vi "Set Exclusions.vi"(4 "Exclude dependent shared libraries":bool, 6 "Exclude dependent packed libraries":bool, 8 "error in (no error)":errorcluster, 9 "Disconnect inline subVIs (T)":bool=TRUE, 10 "Exclusions":T1={"Disconnect type definitions"=FALSE, "Remove unused polymorphic VI instances"=TRUE, "Remove unused members of project libraries"=TRUE, "Modify project library file after removing unused members"=TRUE}, 11 "DLL in":refnum<class "NI_AB_API_DLL.lvclass">) -> (0 "error out":errorcluster, 3 "DLL out":refnum<class "NI_AB_API_DLL.lvclass">)   [LabVIEW 2020, in "NI_AB_API_DLL.lvclass"]
uses:
  <vilib>/AppBuilder/AB_API/DLL/NI_AB_API_DLL.lvclass
  <vilib>/AppBuilder/AB_API/common/AB_API Primary Exclusions.ctl
  <vilib>/AppBuilder/AB_API/Application/NI_AB_API_Application.lvclass
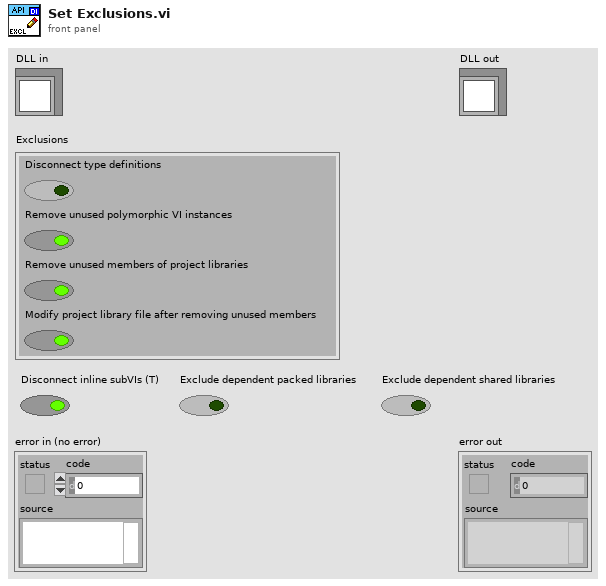
[diagram p1: front panel]
types:
  T1 = typedef "AB_API Primary Exclusions.ctl" = cluster{"Disconnect type definitions":bool, "Remove unused polymorphic VI instances":bool, "Remove unused members of project libraries":bool, "Modify project library file after removing unused members":bool}
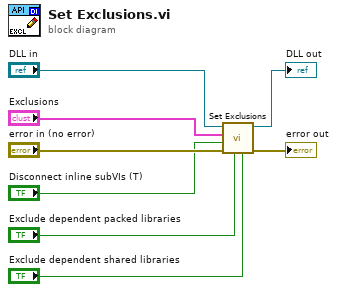
[diagram p0: block diagram]
diagram:
  n1 = call-parent "Set Exclusions.vi"("Exclude dependent shared libraries"="Exclude dependent shared libraries", "Exclude dependent packed libraries"="Exclude dependent packed libraries", "error in (no error)"="error in (no error)", "Disconnect inline subVIs"="Disconnect inline subVIs (T)", "Exclusions"="Exclusions", "Build in"="DLL in") -> ("error out"=→"error out":errorcluster, "Build out"=→"DLL out":refnum<class "NI_AB_API_DLL.lvclass">)  [unwired: 4 in]
